vi "Drug and Drop.vi"() -> ()   [LabVIEW 2015]
panel:
  out "Label.Text":string
  out "Numeric":i32
  out "OK Button 2":bool
  in  "OK Button":bool
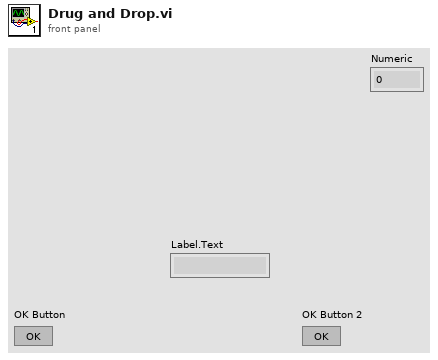
[diagram p1: front panel]
types:
  T1 = cluster{"data name":string, "drag data":variant}[]
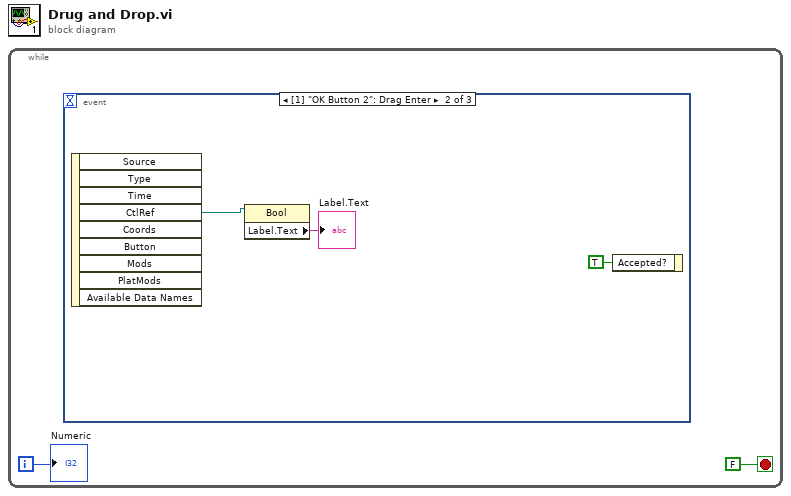
[diagram p0: block diagram]
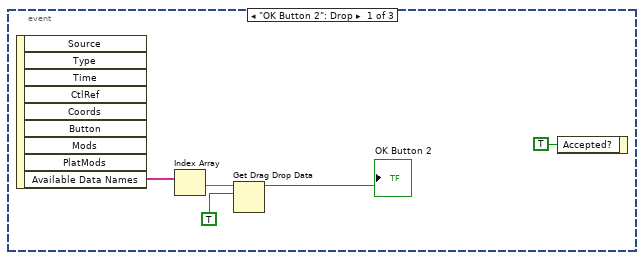
[diagram p2: hidden frame]
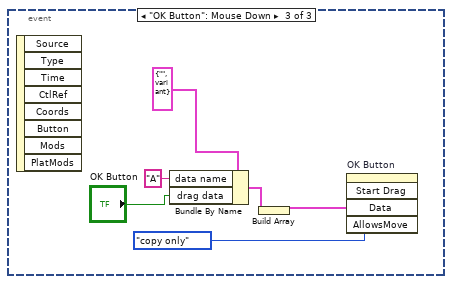
[diagram p3: hidden frame]
diagram:
  n1 = while {
    i -> [w1]
    stop <- FALSE stop-if-true
    n2 = event shown="[1] \"OK Button 2\": Drag Enter" {
      selector: _ -> [_ _ _]
      dyn-events: _ -> [_ _ _]
      timeout: _ -> [_ _ _]
      event "OK Button 2": Drop {
        n3 = event-data() -> ("Available Data Names"=w6:string[])  [unwired: 1 in, 8 out]
        n4 = Index Array(array=w6) -> (element=w5:string)  [unwired: 1 in]
        n5 = Get Drag Drop Data(8:TRUE, 9:w5) -> (3:→"OK Button 2":bool)  [unwired: 1 in, 1 out]
        n6 = event-data("Accepted?"=TRUE) -> ()  [unwired: 1 in, 1 out]
      }
      event "OK Button 2": Drag Enter {
        n7 = event-data() -> ("CtlRef"=w8:refnum<vi>)  [unwired: 1 in, 8 out]
        n8 = property class="Bool"(reference=w8) -> ("Label.Text"=→"Label.Text":string)  [unwired: 1 in, 2 out]
        n9 = event-data("Accepted?"=TRUE) -> ()  [unwired: 1 in, 1 out]
      }
      event "OK Button": Mouse Down {
        n10 = event-data() -> ()  [unwired: 1 in, 8 out]
        n11 = Bundle By Name(cluster=cluster{"data name":string, "drag data":variant} {"data name"="", "drag data"=variant}, "data name"="A", "drag data"="OK Button") -> (w12:cluster{"data name":string, "drag data":variant})
        n12 = Build Array(w12) -> (w11:T1)
        n13 = invoke on="OK Button" class="Bool" method="Start Drag"("Data"=w11, "AllowsMove"=enum32{"copy or move", "copy only", "move only"}."copy only" ("Drag Mode")) -> ()  [unwired: 3 in, 5 out]
      }
    }
    "Numeric" <- w1
  }
